vi "Refresh Files Table.vi"(8 "error in (no error)":errorcluster, 9 "Index":i32=-1, 10 "MulticolumnListbox in":refnum<vi>, 11 "Section Ref in":T1 format="%.0x") -> (0 "error out":errorcluster, 2 "Array":string[][](array[string]), 3 "Section Ref out":T1 format="%.0x")   [LabVIEW 2027, in "Embedded Data Logger System Explorer.lvlib"]
uses:
  Embedded Data Logger System Explorer.lvlib
  <vilib>/NI VeriStand/Custom Device API/Custom Device Item Ref.ctl
  Shared/Constants.vi
  <vilib>/NI VeriStand/Custom Device Tools/Custom Device Utility Library/NI VeriStand - Search for All Items by GUID.vi
  <vilib>/NI VeriStand/Custom Device API/Custom Device API.lvlib
  <vilib>/NI VeriStand/Custom Device Tools/Custom Device Utility Library/Custom Device Utility Library.lvlib
  Shared/Embedded Data Logger Shared.lvlib
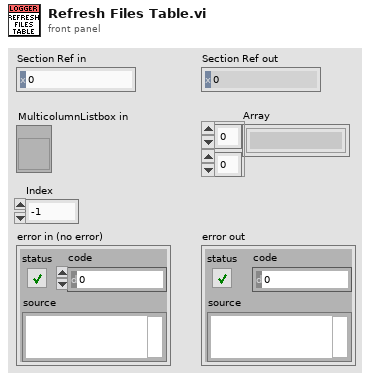
[diagram p1: front panel]
types:
  T1 = typedef "Custom Device API.lvlib/Custom Device Item Ref.ctl" = u64
  T2 = typedef "Custom Device API.lvlib/Custom Device Item Info.ctl" = cluster{"Name":string, "Is Channel":bool, "GUID":string, "Is Waveform":bool}
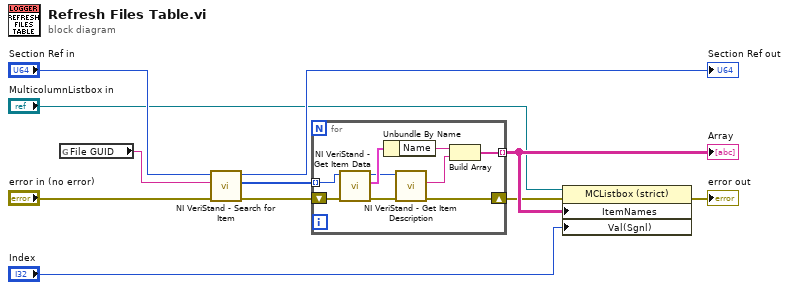
[diagram p0: block diagram]
diagram:
  n1 = global read "Constants.vi" "File GUID"() -> (w11:string)
  n2 = call-poly <vilib>:"NI VeriStand - Search for Item.vi"("error in"="error in (no error)", "Item GUID"=w11, "Section Ref in"="Section Ref in") -> ("error out"=w8:errorcluster, "Item Refs"=w9:T1[], "Section Ref out"=→"Section Ref out":T1)  [unwired: 5 in, 1 out]
  n3 = for {
    tunnel: w9 -> [w19] mode=indexing
    tunnel: [w15] -> w6 mode=indexing
    shift-right: [w14] -> w3
    shift-left: w8 -> [w20]
    n4 = call <vilib>:"NI VeriStand - Get Item Data.vi"("error in (no error)"=w20, "Item Ref in"=w19) -> ("error out"=w12:errorcluster, "Item Info"=w18:T2, "Item Ref out"=w13:T1)  [unwired: 6 in, 1 out]
    n5 = Unbundle By Name(w18) -> ("Name"=w17:string)
    n6 = call <vilib>:"NI VeriStand - Get Item Description.vi"("error in (no error)"=w12, "Item Ref in"=w13) -> ("error out"=w14:errorcluster, "Description"=w16:string)  [unwired: 6 in, 2 out]
    n7 = Build Array(w17, w16) -> (w15:string[])
  }
  "Array" <- w6
  n8 = property on="Property Node" class="MCListbox (strict)"(reference="MulticolumnListbox in", error in=w3, "ItemNames"=w6, "Val(Sgnl)"="Index") -> (error out=→"error out":errorcluster)  [unwired: 1 out]
